vi "controlValuesManual.vi"(8 "error in (no error)":errorcluster) -> (0 "error out":errorcluster, 3 "controlBufferOut":sgl[](array[numeric]))   [LabVIEW 2016]
uses:
  <userlib>/cameraLibrary/cameraLibrary.lvlib
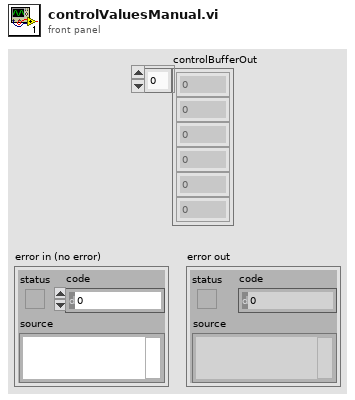
[diagram p1: front panel]
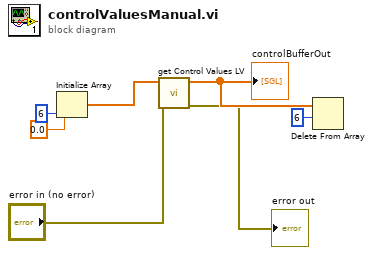
[diagram p0: block diagram]
diagram:
  n1 = Initialize Array(sgl 0.0 ("element"), 6 ("dimension size")) -> (w7:sgl[])
  n2 = call <userlib>:"get Control Values LV.vi"("error in (no error)"="error in (no error)", "controlBufferIn"=w7) -> ("error out"=→"error out":errorcluster, "controlBufferOut"=w4:sgl[])  [unwired: 8 in]
  "controlBufferOut" <- w4
  n3 = Delete From Array(array=w4, length=6) -> ()  [unwired: 1 in, 2 out]
